vi "Send Command.vi"(7 "Command":string, 8 "error in (no error)":errorcluster, 11 "connection ID":refnum<k5>) -> (0 "error out":errorcluster, 3 "connection ID out":refnum<k5>)   [LabVIEW 2019, in "ACSVcontrol-driver.lvlib"]
doc: "Send command trhough TCP."
uses:
  ACSVcontrol-driver.lvlib
  Type definitions/Instruction.ctl
  Type definitions/Debug data.ctl
  Globals.vi
  <vilib>/Utility/error.llb/Error Cluster From Error Code.vi
  <vilib>/ErrorRing/Error Ring.xnode
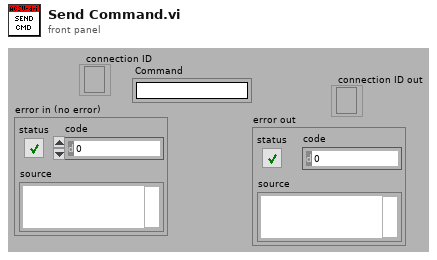
[diagram p1: front panel]
types:
  T1 = typedef "ACSVcontrol-driver.lvlib/Timeouts.ctl" = cluster{"TCP Read & Write (ms)":i32, "Sensors readout":i32, "PJVS setup":i32, "Nullmeter readout":i32, "Multiplexer setup":i32, "57XX setup":i32, "Generator setup":i32, "Synthesizer setup":i32, "Sampler readout":i32}
  T2 = typedef "ACSVcontrol-driver.lvlib/Instruction.ctl" = enum16{"dummy - do not use", "Send Command", "Read Result", "Ask Status"}
  T3 = typedef "ACSVcontrol-driver.lvlib/Debug data.ctl" = cluster{"Time Stamp":timestamp, "Data":string, "Write":bool, "Call chain":string[], "Error after":errorcluster}
  T4 = typedef "ACSVcontrol-driver.lvlib/Debug status.ctl" = enum16{"No change", "Off", "On"}
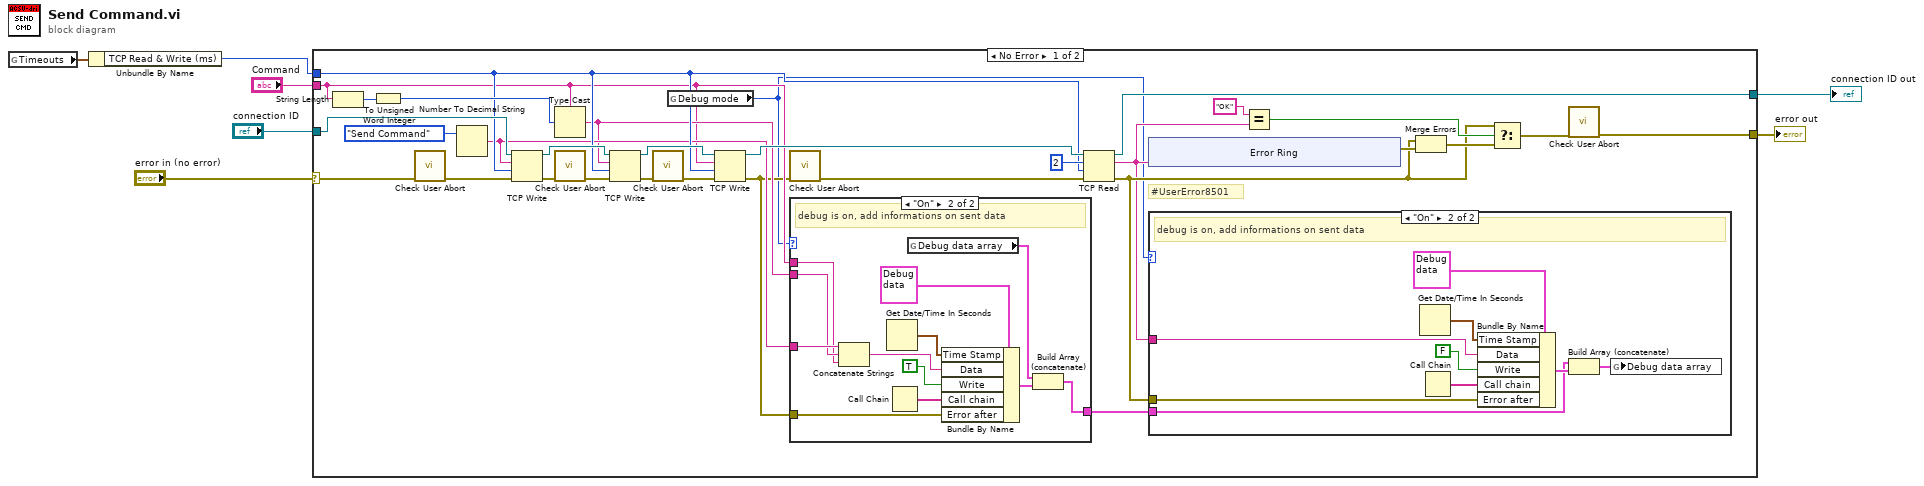
[diagram p0: block diagram]
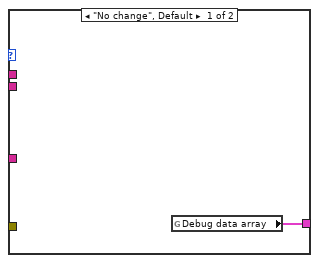
[diagram p3: hidden frame]
diagram:
  n1 = global read "Globals.vi" "Timeouts"() -> (w1:T1)
  n2 = Unbundle By Name(w1) -> ("TCP Read & Write (ms)"=w2:i32)
  n3 = case shown="No Error" "error in (no error)" {
    selector: "error in (no error)" -> [w17 w69]
    tunnel: [w31 w68] -> w5
    tunnel: [w18 w69] -> w6
    tunnel: "connection ID" -> [w30 w68]
    tunnel: "Command" -> [w13 _]
    tunnel: w2 -> [w29 _]
    frame No Error {
      # "#UserError8501"
      n4 = String Length(string=w13) -> (length=w33:i32)
      n5 = To Unsigned Word Integer(number=w33) -> (unsigned 16bit integer=w32:u16)
      n6 = call "Check User Abort.vi"("error in (no error)"=w17) -> ("error out"=w16:errorcluster)  [unwired: 10 in]
      n7 = Number To Decimal String(number=Instruction."Send Command" ("Instruction")) -> (decimal integer string=w15:string)  [unwired: 1 in]
      n8 = TCP Write(connection ID=w30, data in=w15, error in (no error)=w16, 9:w29) -> (connection ID out=w38:refnum<k5>, error out=w24:errorcluster)  [unwired: 1 out]
      n9 = Type Cast(type=w13, x=w32) -> (*(type *) &x=w14:string)
      n10 = call "Check User Abort.vi"("error in (no error)"=w24) -> ("error out"=w23:errorcluster)  [unwired: 10 in]
      n11 = TCP Write(connection ID=w38, data in=w14, error in (no error)=w23, 9:w29) -> (connection ID out=w37:refnum<k5>, error out=w22:errorcluster)  [unwired: 1 out]
      n12 = call "Check User Abort.vi"("error in (no error)"=w22) -> ("error out"=w21:errorcluster)  [unwired: 10 in]
      n13 = global read "Globals.vi" "Debug mode"() -> (w8:T4)
      n14 = TCP Write(connection ID=w37, data in=w13, error in (no error)=w21, 9:w29) -> (connection ID out=w34:refnum<k5>, error out=w12:errorcluster)  [unwired: 1 out]
      n15 = call "Check User Abort.vi"("error in (no error)"=w12) -> ("error out"=w20:errorcluster)  [unwired: 10 in]
      n16 = case shown="\"On\"" w8 {
        tunnel: w15 -> [_ w56]
        tunnel: w14 -> [_ w55]
        tunnel: w13 -> [_ w54]
        tunnel: w12 -> [_ w50]
        tunnel: [w48 w49] -> w9
        frame "No change", Default {
          n17 = global read "Globals.vi" "Debug data array"() -> (w48:T3[])
        }
        frame "On" {
          # "debug is on, add informations on sent data"
          n18 = Concatenate Strings(w56, w55, w54) -> (w53:string)
          n19 = Get Date/Time In Seconds() -> (seconds since 1Jan1904=w59:timestamp)
          n20 = Call Chain() -> (call chain=w58:string[])
          n21 = global read "Globals.vi" "Debug data array"() -> (w52:T3[])
          n22 = Bundle By Name(cluster=T3 {"Time Stamp"=timestamp(0 s since 1904-01-01), "Data"="", "Write"=FALSE, "Call chain"=[], "Error after"={"status"=FALSE, "code"=0, "source"=""}} ("Debug data"), "Time Stamp"=w59, "Data"=w53, "Write"=TRUE ("Sent"), "Call chain"=w58, "Error after"=w50) -> (w51:T3)
          n23 = Build Array (concatenate)(w52, w51) -> (w49:T3[])
        }
      }
      n24 = TCP Read(connection ID=w34, bytes to read=2, error in (no error)=w20, 9:w29) -> (connection ID out=w31:refnum<k5>, data out=w10:string, error out=w11:errorcluster)  [unwired: 1 in]
      n25 = xnode "Error Ring"("parameter 0"=w10) -> ("error out"=w27:errorcluster)
      n26 = case shown="\"On\"" w8 {
        tunnel: w11 -> [_ w41]
        tunnel: w10 -> [_ w40]
        tunnel: w9 -> [_ w39]
        frame "No change", Default {
        }
        frame "On" {
          # "debug is on, add informations on sent data"
          n27 = Get Date/Time In Seconds() -> (seconds since 1Jan1904=w46:timestamp)
          n28 = Call Chain() -> (call chain=w45:string[])
          n29 = Bundle By Name(cluster=T3 {"Time Stamp"=timestamp(0 s since 1904-01-01), "Data"="", "Write"=FALSE, "Call chain"=[], "Error after"={"status"=FALSE, "code"=0, "source"=""}} ("Debug data"), "Time Stamp"=w46, "Data"=w40, "Write"=FALSE ("Sent"), "Call chain"=w45, "Error after"=w41) -> (w43:T3)
          n30 = Build Array (concatenate)(w39, w43) -> (w42:T3[])
          n31 = global write "Globals.vi" "Debug data array"(w42) -> ()
        }
      }
      n32 = Equal?(x="OK", y=w10) -> (x = y?=w28:bool)
      n33 = Merge Errors(w11, w27) -> (w26:errorcluster)
      n34 = Select(t=w11, s=w28, f=w26) -> (s? t:f=w19:errorcluster)
      n35 = call "Check User Abort.vi"("error in (no error)"=w19) -> ("error out"=w18:errorcluster)  [unwired: 10 in]
    }
    frame Error {
    }
  }
  "error out" <- w6
  "connection ID out" <- w5
